vi "Login.vi"() -> ()   [LabVIEW 2018]
panel:
  out "Login correct？":bool
  in  "Close":bool
  in  "Login":bool
  in  "Code":string
  in  "User":string
  in  "ctl":bool
  # "C&M SERVO PRESS SOFTWARE SYSTEM"
  # "User："
  # "Code："
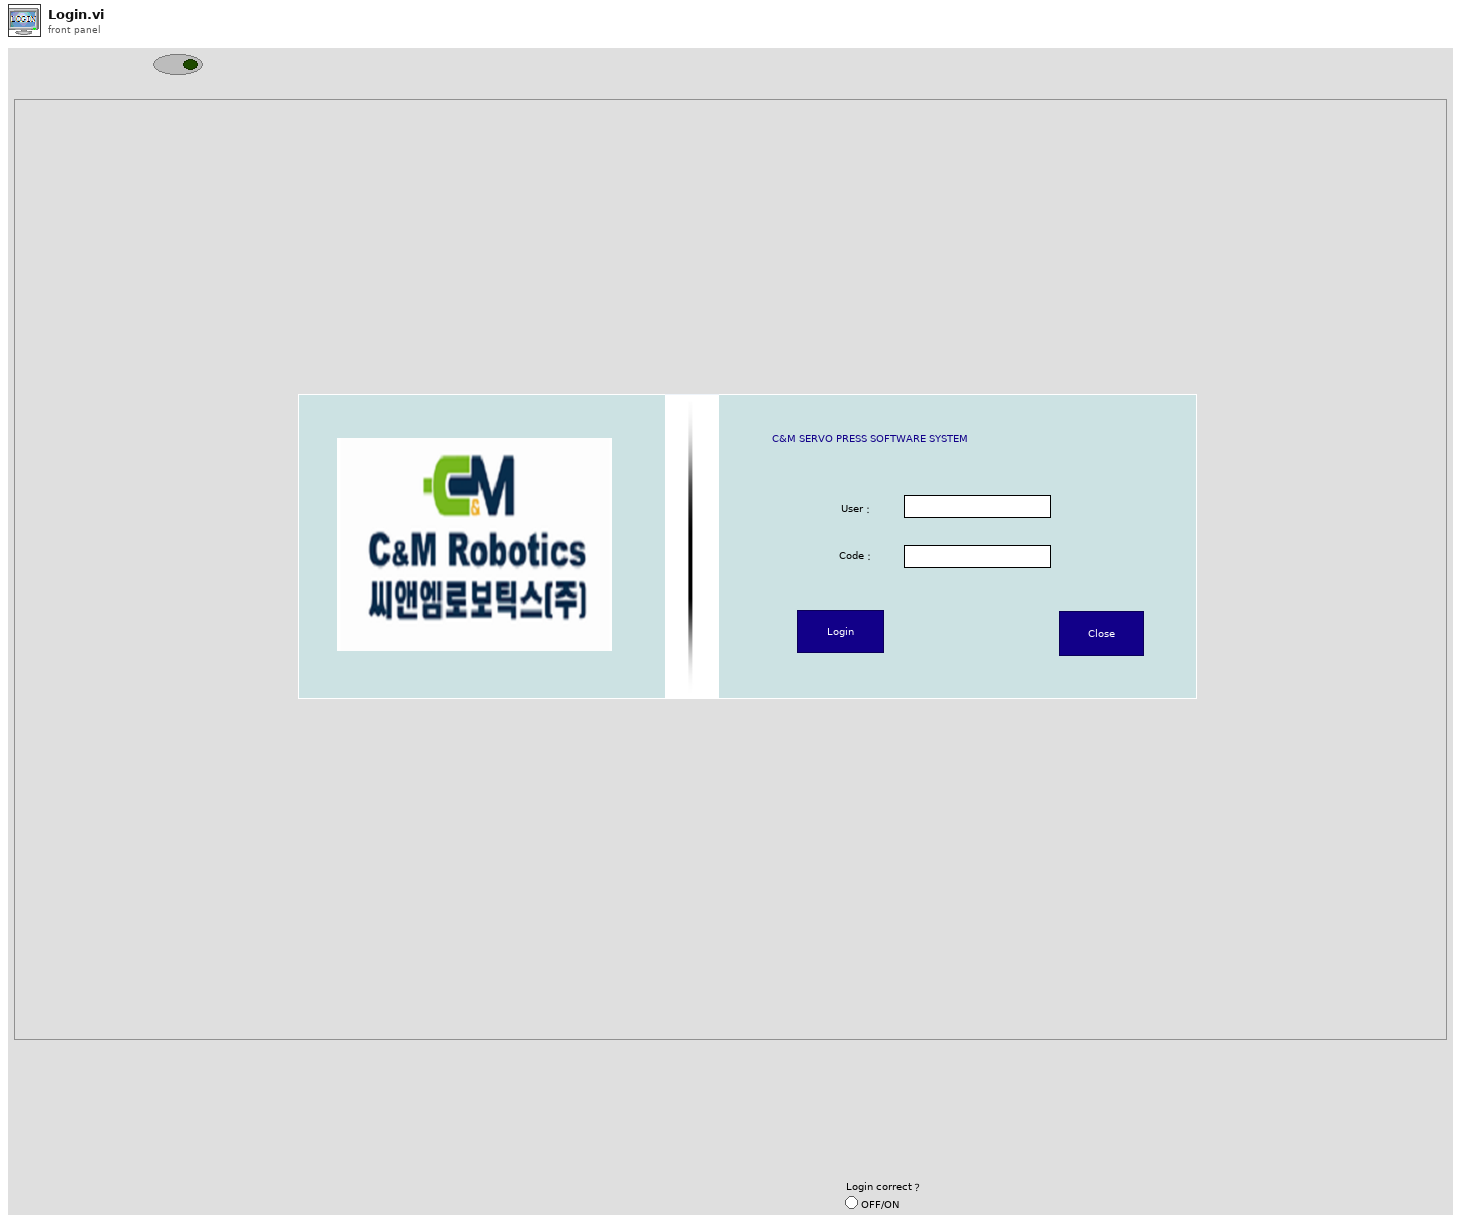
[diagram p1: front panel]
types:
  T1 = enum8{"Enabled", "Disabled", "Disabled and Grayed Out"}
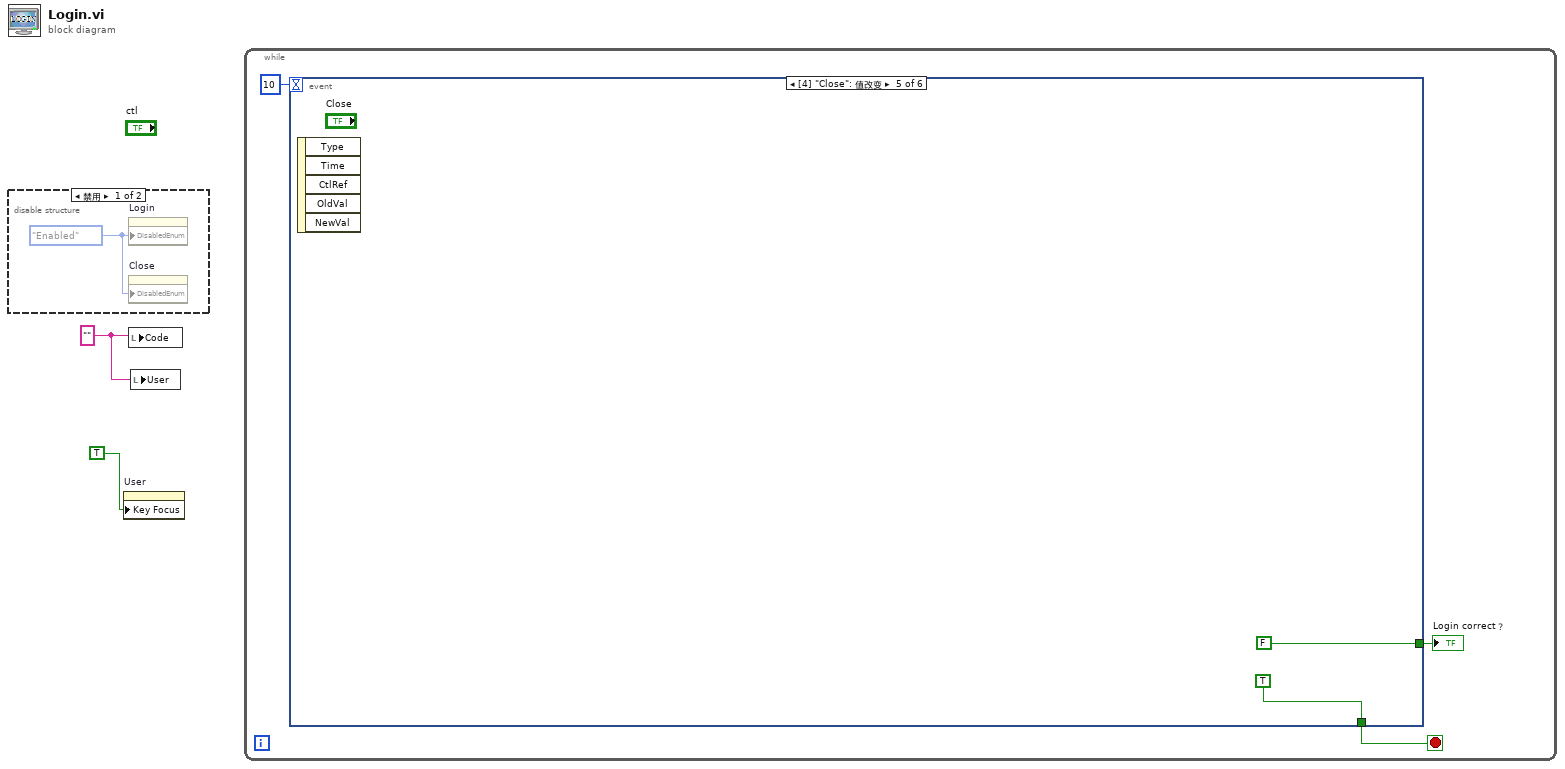
[diagram p0: block diagram]
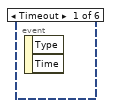
[diagram p3: hidden frame]
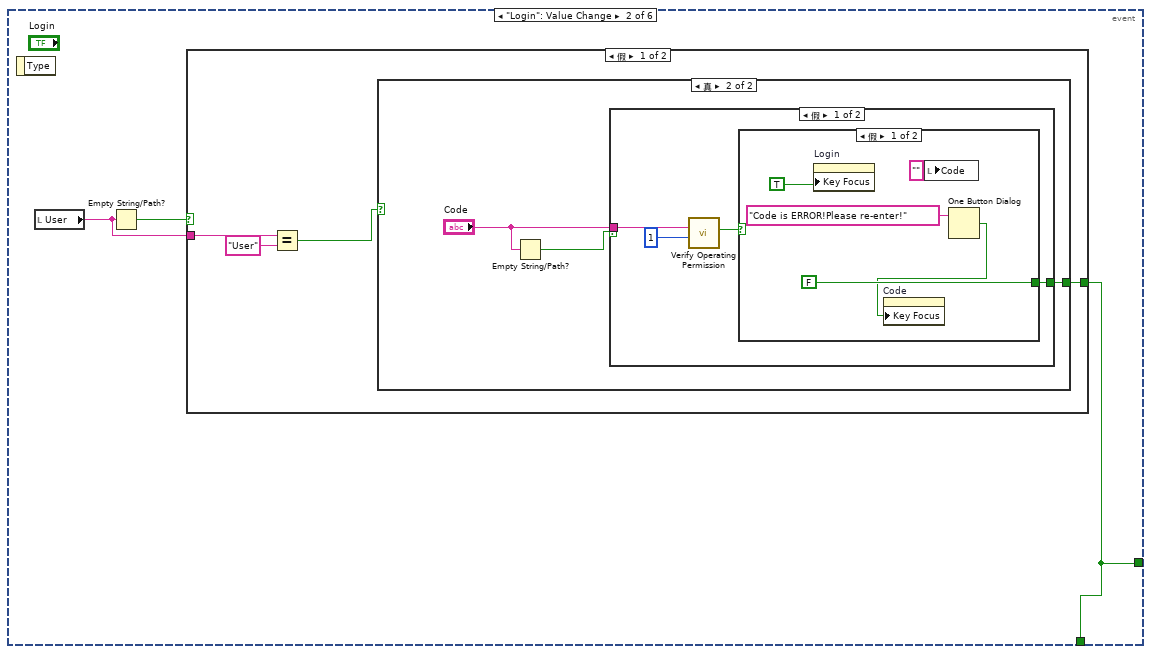
[diagram p4: hidden frame]
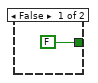
[diagram p5: hidden frame]
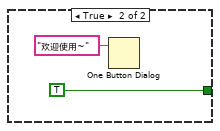
[diagram p6: hidden frame]
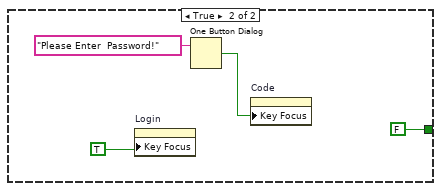
[diagram p7: hidden frame]
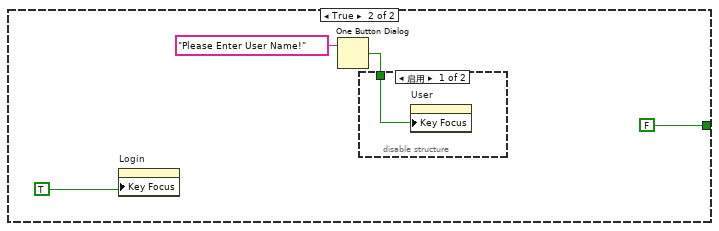
[diagram p8: hidden frame]
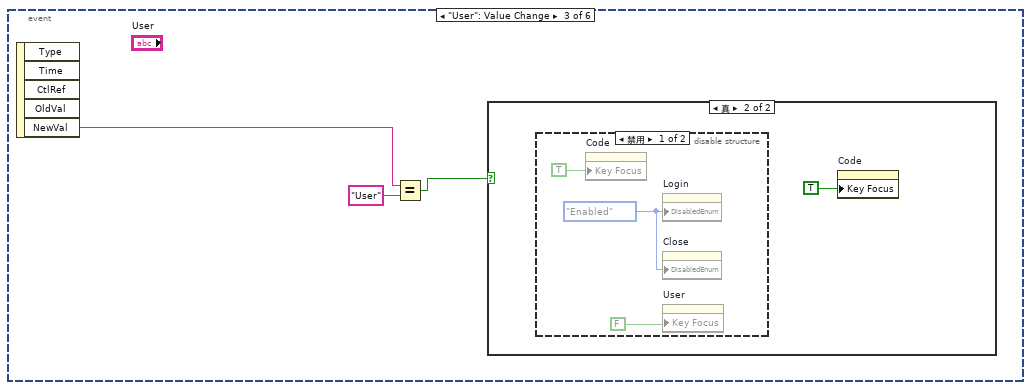
[diagram p10: hidden frame]
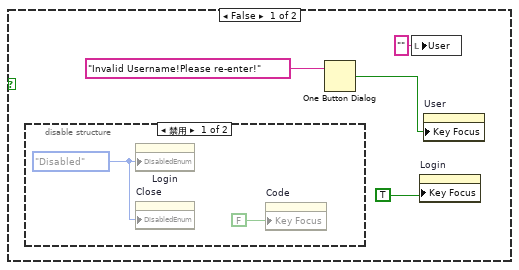
[diagram p11: hidden frame]
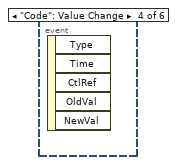
[diagram p14: hidden frame]
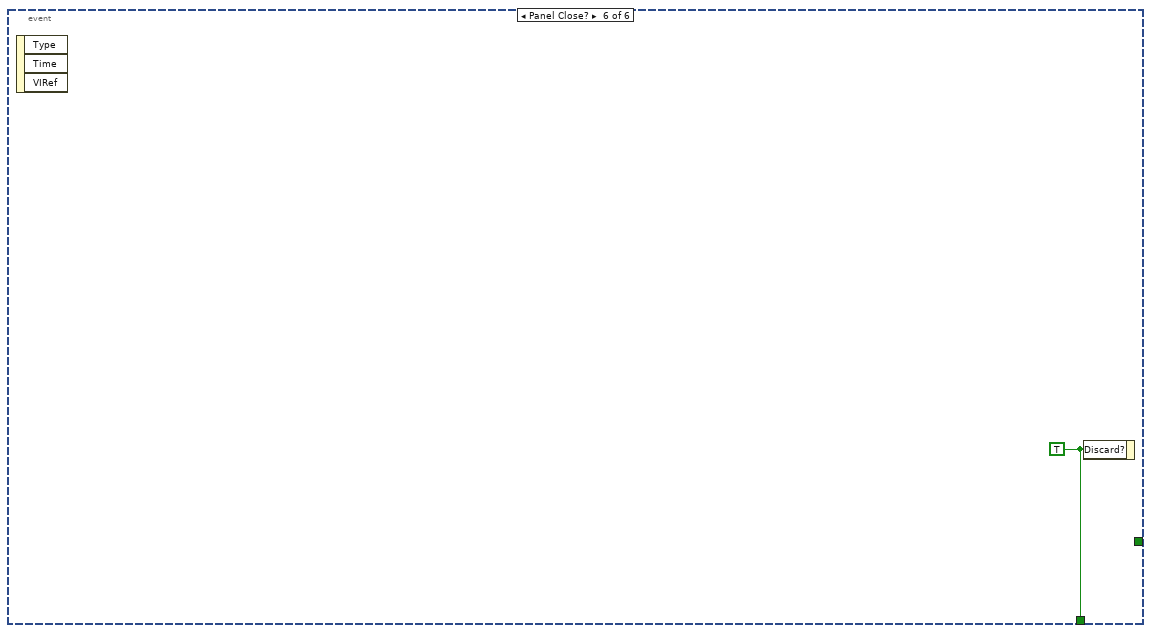
[diagram p15: hidden frame]
diagram:
  w2 = "" ("y")
  n1 = disable-structure shown="禁用" {
    frame Disabled {
      w3 = T1."Enabled" ("禁用")
      n2 = property on="Login" class="Bool"("DisabledEnum"=w3) -> ()  [unwired: 2 in, 2 out]
      n3 = property on="Close" class="Bool"("DisabledEnum"=w3) -> ()  [unwired: 2 in, 2 out]
    }
    frame Enabled {
    }
  }
  n4 = property on="User" class="Str"("Key Focus"=TRUE ("键选中")) -> ()  [unwired: 2 in, 2 out]
  n5 = local write "Code"(w2) -> ()
  n6 = local write "User"(w2) -> ()
  n7 = while {
    stop <- w5 stop-if-true
    n8 = event shown="[4] \"Close\": 值改变" {
      selector: _ -> [_ _ _ _ _ _]
      dyn-events: _ -> [_ _ _ _ _ _]
      timeout: 10 -> [_ _ _ _ _ _]
      tunnel: [_ w9 _ _ TRUE ("放弃？") w53] -> w5
      tunnel: [_ w9 _ _ FALSE ("放弃？") _] -> w4
      event Timeout {
        n9 = event-data() -> ()  [unwired: 1 in, 2 out]
      }
      event "Login": Value Change {
        n10 = event-data() -> ()  [unwired: 1 in, 1 out]
        n11 = local read "User"() -> (w7:string)
        n12 = Empty String/Path?(string/path=w7) -> (empty?=w8:bool)
        n13 = case shown="假" w8 {
          tunnel: [w13 FALSE ("放弃？")] -> w9
          tunnel: w7 -> [w12 _]
          frame False {
            n14 = Equal?(x=w12, y="User") -> (x = y?=w10:bool)
            n15 = case shown="真" w10 {
              tunnel: [FALSE ("放弃？") w17] -> w13
              frame False {
              }
              frame True {
                n16 = Empty String/Path?(string/path="Code") -> (empty?=w15:bool)
                n17 = case shown="假" w15 {
                  tunnel: "Code" -> [w20 _]
                  tunnel: [w18 FALSE ("放弃？")] -> w17
                  frame False {
                    n18 = call "Verify Operating Permission.vi"("权限选择"=1, "密码"=w20) -> ("验证成功"=w19:bool)  [unwired: 9 in]
                    n19 = case shown="假" w19 {
                      tunnel: [FALSE ("OK") TRUE ("放弃？")] -> w18
                      frame False {
                        n20 = property on="Login" class="Bool"("Key Focus"=TRUE ("键选中")) -> ()  [unwired: 2 in, 2 out]
                        n21 = local write "Code"("" ("Code")) -> ()
                        n22 = One Button Dialog(message="Code is ERROR!Please re-enter!" ("消息")) -> (true=w24:bool)  [unwired: 1 in]
                        n23 = property on="Code" class="Str"("Key Focus"=w24) -> ()  [unwired: 2 in, 2 out]
                      }
                      frame True {
                        n24 = One Button Dialog(message="欢迎使用~" ("消息")) -> ()  [unwired: 1 in, 1 out]
                      }
                    }
                  }
                  frame True {
                    n25 = property on="Login" class="Bool"("Key Focus"=TRUE ("键选中")) -> ()  [unwired: 2 in, 2 out]
                    n26 = One Button Dialog(message="Please Enter  Password!" ("消息")) -> (true=w30:bool)  [unwired: 1 in]
                    n27 = property on="Code" class="Str"("Key Focus"=w30) -> ()  [unwired: 2 in, 2 out]
                  }
                }
              }
            }
          }
          frame True {
            n28 = property on="Login" class="Bool"("Key Focus"=TRUE ("键选中")) -> ()  [unwired: 2 in, 2 out]
            n29 = One Button Dialog(message="Please Enter User Name!" ("消息")) -> (true=w34:bool)  [unwired: 1 in]
            n30 = disable-structure shown="启用" {
              disable-tunnel: w34 -> [w37 _]
              frame Enabled {
                n31 = property on="User" class="Str"("Key Focus"=w37) -> ()  [unwired: 2 in, 2 out]
              }
              frame Disabled {
              }
            }
          }
        }
      }
      event "User": Value Change {
        n32 = event-data() -> ("NewVal"=w39:string)  [unwired: 1 in, 4 out]
        n33 = Equal?(x=w39, y="User") -> (x = y?=w38:bool)
        n34 = case shown="真" w38 {
          frame False {
            n35 = disable-structure shown="禁用" {
              frame Disabled {
                w46 = T1."Disabled" ("禁用")
                n36 = property on="Login" class="Bool"("DisabledEnum"=w46) -> ()  [unwired: 2 in, 2 out]
                n37 = property on="Close" class="Bool"("DisabledEnum"=w46) -> ()  [unwired: 2 in, 2 out]
                n38 = property on="Code" class="Str"("Key Focus"=FALSE ("键选中")) -> ()  [unwired: 2 in, 2 out]
              }
              frame Enabled {
              }
            }
            n39 = One Button Dialog(message="Invalid Username!Please re-enter!" ("消息")) -> (true=w43:bool)  [unwired: 1 in]
            n40 = local write "User"("" ("User")) -> ()
            n41 = property on="Login" class="Bool"("Key Focus"=TRUE ("键选中")) -> ()  [unwired: 2 in, 2 out]
            n42 = property on="User" class="Str"("Key Focus"=w43) -> ()  [unwired: 2 in, 2 out]
          }
          frame True {
            n43 = disable-structure shown="禁用" {
              frame Disabled {
                w50 = T1."Enabled" ("禁用")
                n44 = property on="Code" class="Str"("Key Focus"=TRUE ("键选中")) -> ()  [unwired: 2 in, 2 out]
                n45 = property on="Login" class="Bool"("DisabledEnum"=w50) -> ()  [unwired: 2 in, 2 out]
                n46 = property on="Close" class="Bool"("DisabledEnum"=w50) -> ()  [unwired: 2 in, 2 out]
                n47 = property on="User" class="Str"("Key Focus"=FALSE ("键选中")) -> ()  [unwired: 2 in, 2 out]
              }
              frame Enabled {
              }
            }
            n48 = property on="Code" class="Str"("Key Focus"=TRUE ("键选中")) -> ()  [unwired: 2 in, 2 out]
          }
        }
      }
      event "Code": Value Change {
        n49 = event-data() -> ()  [unwired: 1 in, 5 out]
      }
      event "Close": Value Change {
        n50 = event-data() -> ()  [unwired: 1 in, 5 out]
      }
      event Panel Close? {
        w53 = TRUE ("放弃？")
        n51 = event-data() -> ()  [unwired: 1 in, 3 out]
        n52 = event-data("Discard?"=w53) -> ()  [unwired: 1 in, 1 out]
      }
    }
    "Login correct？" <- w4
  }
